vi "wait on results.vi"(8 "error in":errorcluster, 9 "timeout per element":i32=-1, 10 "count":i32=1, 11 "queue reporter in":refnum<class "queue reporter.lvclass">) -> (0 "error out":errorcluster, 2 "results":refnum<class "result.lvclass">[](array[class]), 3 "queue reporter out":refnum<class "queue reporter.lvclass">)   [LabVIEW 2013, in "queue reporter.lvclass"]
uses:
  queue reporter.lvclass
  result/result.lvclass
  queue reporter.lvclass/queue reporter.ctl
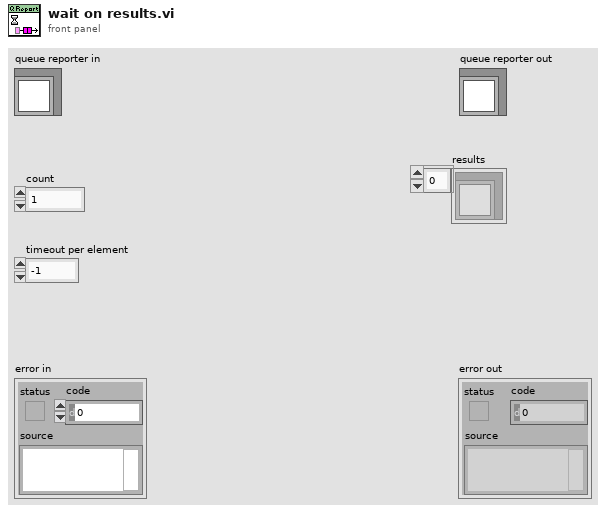
[diagram p1: front panel]
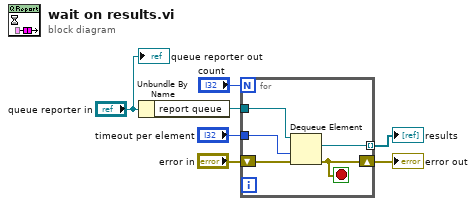
[diagram p0: block diagram]
diagram:
  n1 = Unbundle By Name("queue reporter in") -> ("report queue"=w4:refnum<queue>)
  n2 = for {
    N: "count" -> [_]
    shift-right: [w11] -> w5
    shift-left: "error in" -> [w12]
    tunnel: w4 -> [w10]
    tunnel: [w9] -> w3 mode=indexing
    tunnel: "timeout per element" -> [w8]
    stop <- w11 stop-if-true
    n3 = Dequeue Element(queue=w10, timeout in ms (-1)=w8, error in (no error)=w12) -> (element=w9:refnum<class "result.lvclass">, error out=w11:errorcluster)  [unwired: 2 out]
  }
  "error out" <- w5
  "results" <- w3
  "queue reporter out" <- "queue reporter in"
